vi "UE9 Single AIN Example.vi"() -> ()   [LabVIEW 2021]
panel:
  out "Error Message":string
  in  "Resolution":i32=12
  in  "AIN Range":u16(ring) items=["LJ_rgBIP5V", "LJ_rgUNI5V", "LJ_rgUNI2P5V", "LJ_rgUNI1P25V", "LJ_rgUNIP625V"]
  out "error out":errorcluster
  out "Value Read":dbl format="%.6f"
  in  "Channel #":i32
  # "Aquires 1 analog input channel from the first found UE9 over USB."
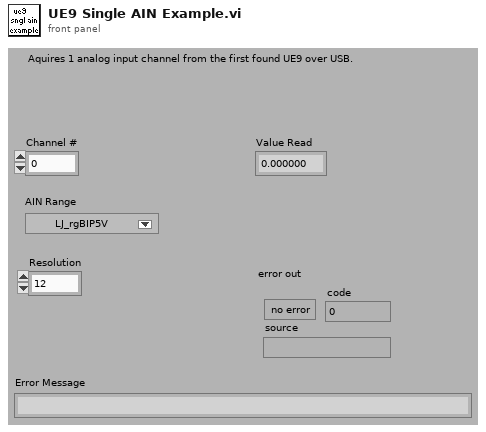
[diagram p1: front panel]
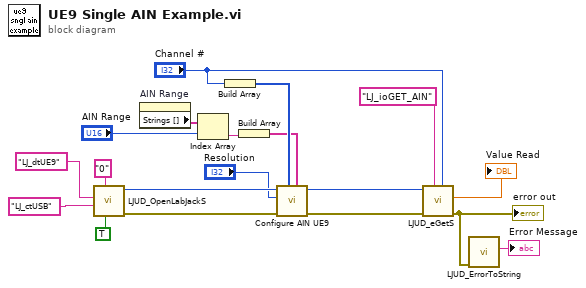
[diagram p0: block diagram]
diagram:
  n1 = call "LJUD_OpenLabJackS.vi"("FirstFound"=TRUE, "Address"="0", "ConnectionType"="LJ_ctUSB", "DeviceType"="LJ_dtUE9") -> ("error out"=w18:errorcluster, "Handle"=w19:i32)  [unwired: 5 in, 1 out]
  n2 = property on="AIN Range" class="Ring (strict)"() -> ("Strings []"=w5:string[])  [unwired: 2 in, 2 out]
  n3 = Index Array(array=w5, index="AIN Range") -> (element=w3:string)
  n4 = Build Array("Channel #") -> (w7:i32[])
  n5 = Build Array(w3) -> (w2:string[])
  n6 = call "Configure AIN UE9.vi"("Ranges"=w2, "Channels"=w7, "error in"=w18, "Resolution"="Resolution", "Handle In"=w19) -> ("error out"=w17:errorcluster, "Handle Out"=w16:i32)  [unwired: 5 in]
  n7 = call "LJUD_eGetS.vi"("Channel"="Channel #", "IOType"="LJ_ioGET_AIN", "error in"=w17, "Handle In"=w16) -> ("error out"=w11:errorcluster, "Value Read"=→"Value Read":dbl)  [unwired: 5 in, 1 out]
  "error out" <- w11
  n8 = call "LJUD_ErrorToString.vi"("error in"=w11) -> ("String"=→"Error Message":string)  [unwired: 10 in]
